vi "Harvest_Folder_Client.vi"(4 "Get all Server Files":bool, 5 "Check Updates on Server?":bool, 6 "Archive Files?":bool, 7 "Folder to Harvest":path=path "/Lacie_20/EnFlo_Data/Andrew_Burt/Results") -> (0 "error out":errorcluster, 1 "Folder contents changed?":bool, 2 "Files to Pull From Server":path[](array[path]), 3 "Files to Push to Server":path[](array[path]))   [LabVIEW 2013]
uses:
  Sub VIs/Harvest_Global.vi
  Anemometry/Anemometry Sub Vis/Globals/Preference_global.vi
  Anemometry/Anemometry Sub Vis/Globals/Constants_global.vi
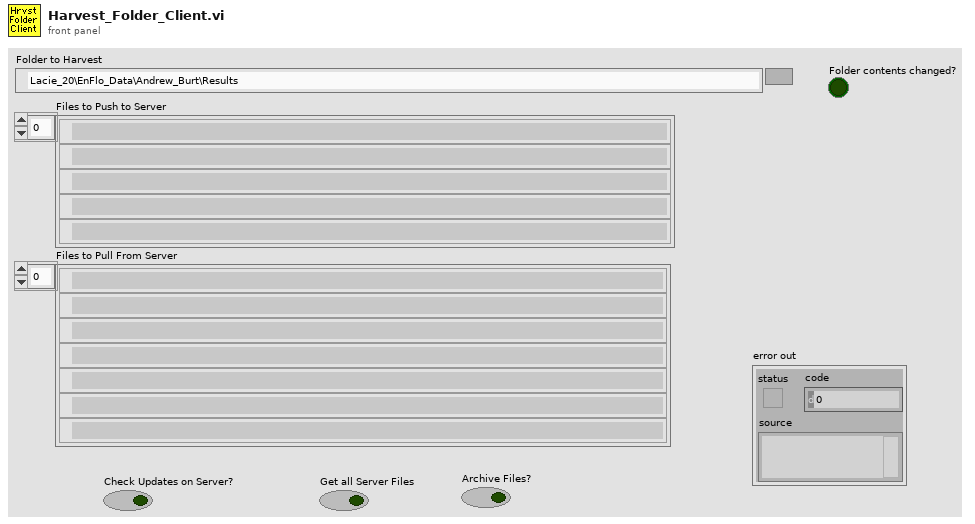
[diagram p1: front panel]
types:
  T1 = typedef "Server_Comms.ctl" = enum16{"Server Link Healthy", "Do Not Link To Server"}
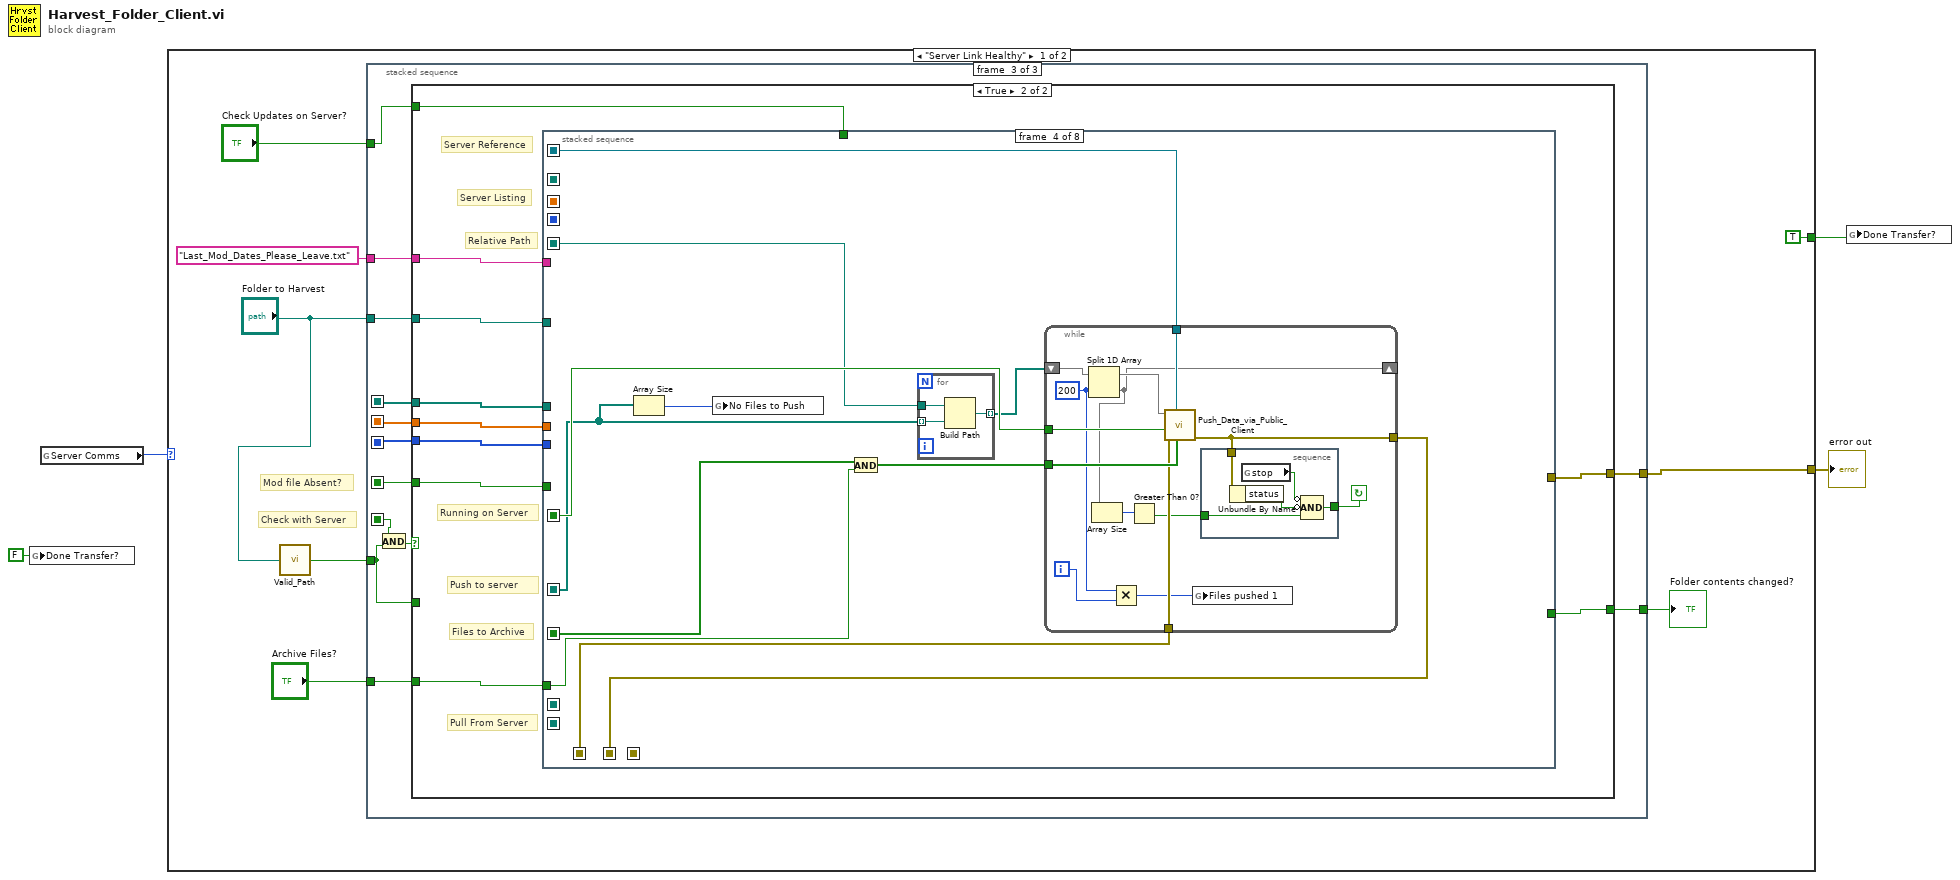
[diagram p0: block diagram]
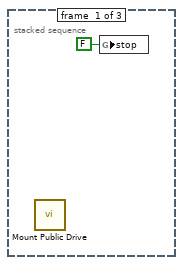
[diagram p2: hidden frame]
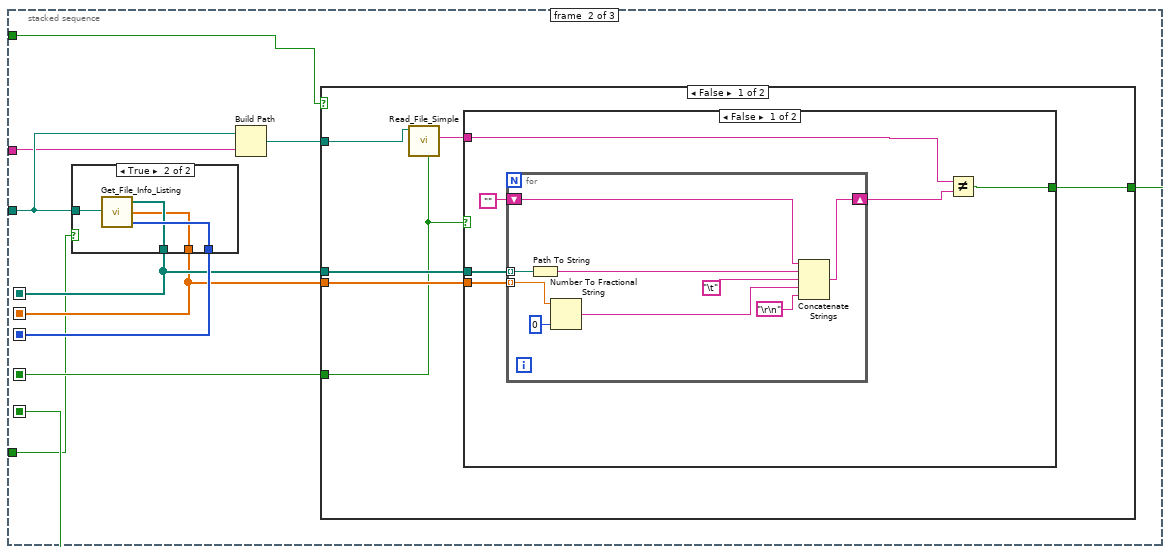
[diagram p3: hidden frame]
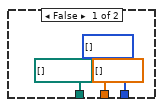
[diagram p4: hidden frame]
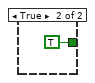
[diagram p5: hidden frame]
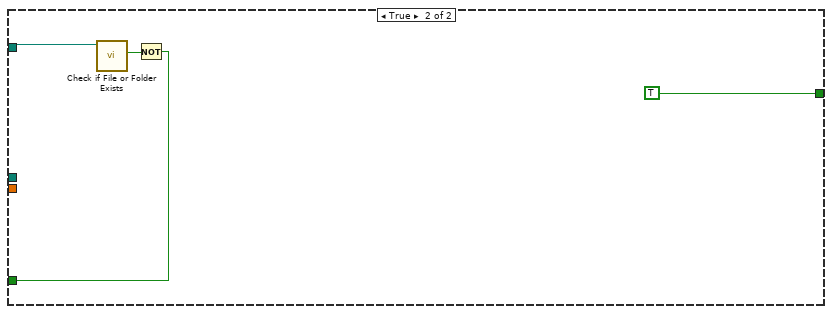
[diagram p6: hidden frame]
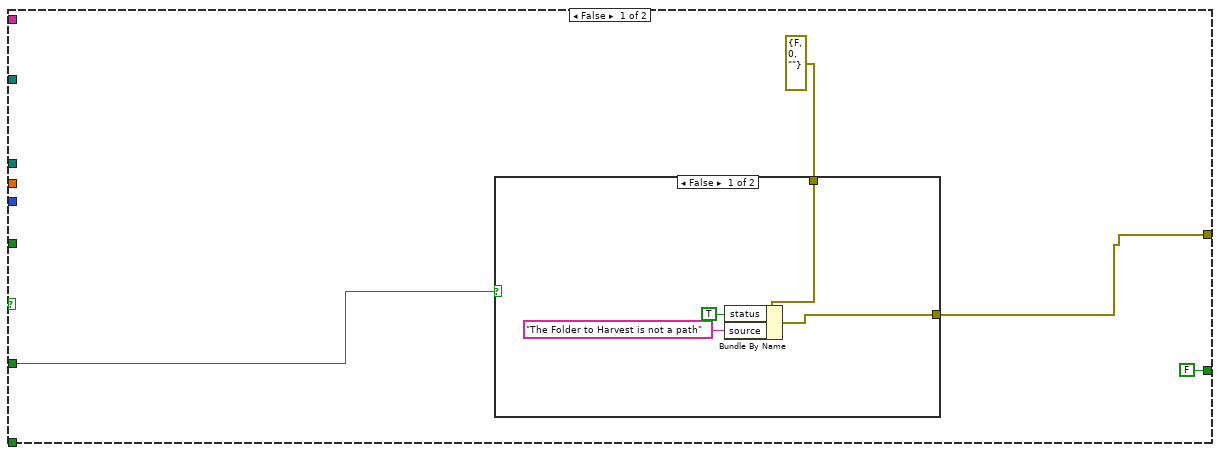
[diagram p7: hidden frame]
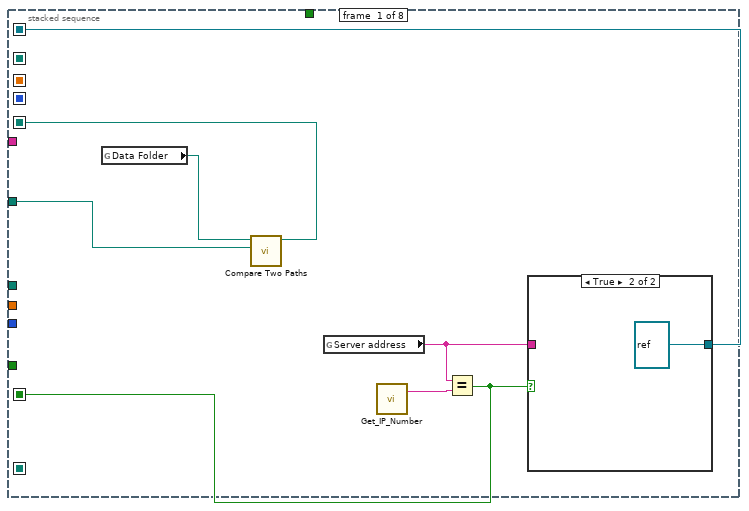
[diagram p9: hidden frame]
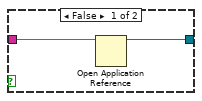
[diagram p10: hidden frame]
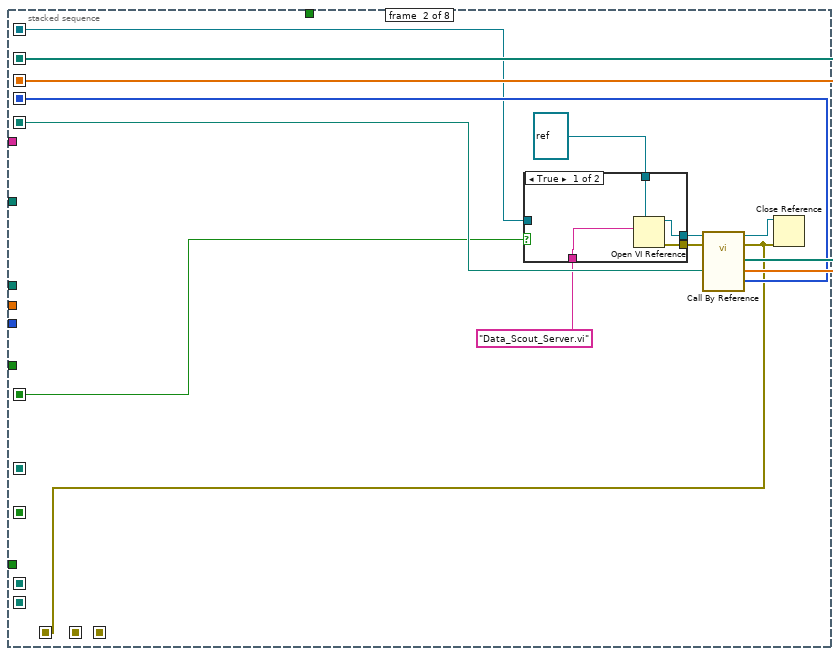
[diagram p11: hidden frame]
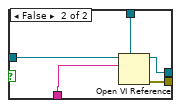
[diagram p12: hidden frame]
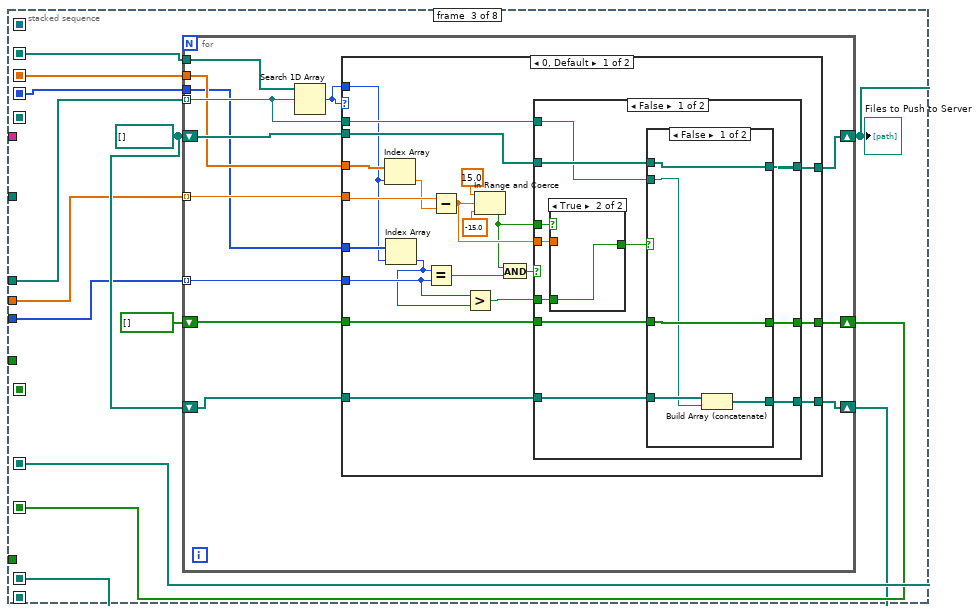
[diagram p13: hidden frame]
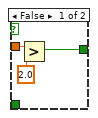
[diagram p14: hidden frame]
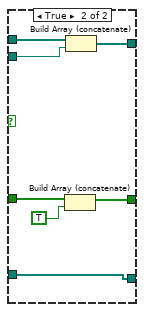
[diagram p15: hidden frame]
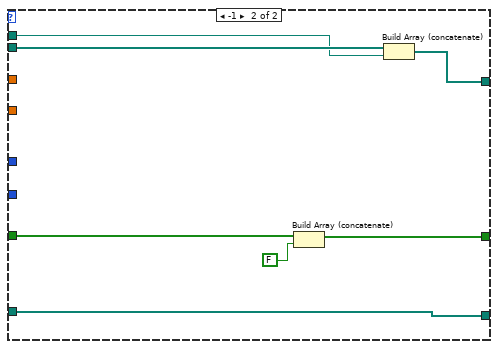
[diagram p17: hidden frame]
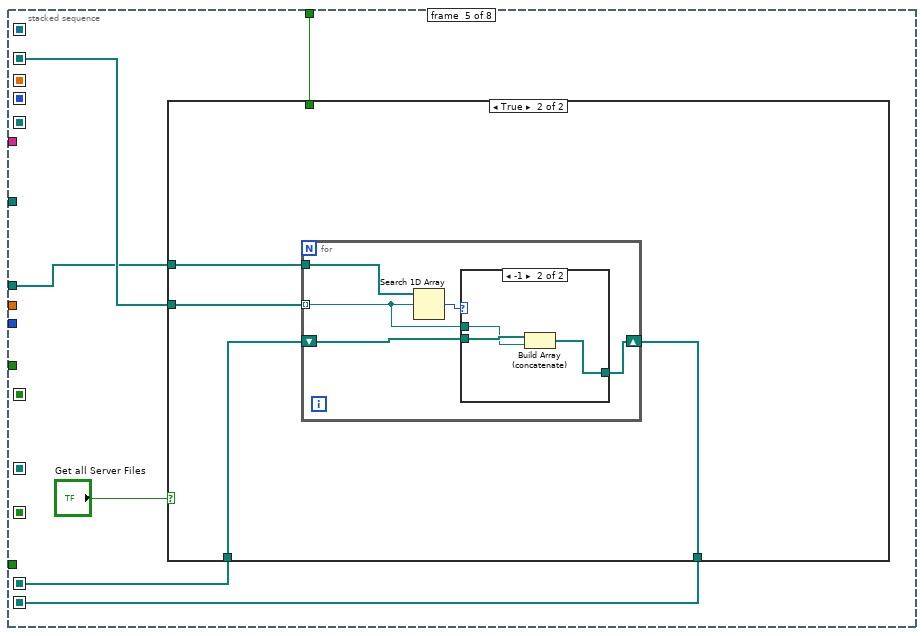
[diagram p18: hidden frame]
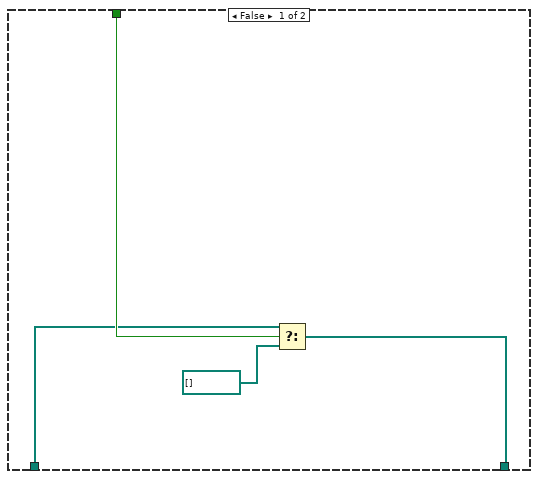
[diagram p19: hidden frame]
diagram:
  n1 = global write "Harvest_Global.vi" "Done Transfer?"(FALSE ("Done Transfer?")) -> ()
  n2 = global read "Preference_global.vi" "Server Comms"() -> (w4:T1)
  n3 = case shown="\"Server Link Healthy\"" w4 {
    tunnel: [w6 w324] -> w3
    tunnel: [TRUE ("Done Transfer?") TRUE ("Done Transfer?")] -> w1
    frame "Server Link Healthy" {
      # "Mod file Absent?"
      # "Check with Server"
      n4 = call "Valid_Path.vi"("Filename"="Folder to Harvest") -> ("Valid Path?"=w9:bool)
      n5 = stacked-sequence {
        seq-local: [_ w22 _] -> [_ _ w68]
        seq-local: [_ w21 _] -> [_ _ w67]
        seq-local: [_ w23 _] -> [_ _ w66]
        seq-local: [_ w20 _] -> [_ _ w61]
        seq-local: [_ w19 _] -> [_ _ w62]
        tunnel: "Folder to Harvest" -> [_ w18 w69]
        tunnel: "Last_Mod_Dates_Please_Leave.txt" ("name or relative path") -> [_ w17 w65]
        tunnel: [_ _ w64] -> w6
        tunnel: [_ _ w63] -> w11
        tunnel: w9 -> [_ w15 w59]
        tunnel: "Archive Files?" -> [_ _ w58]
        tunnel: "Check Updates on Server?" -> [_ w14 w57]
        frame #0 {
          n6 = call "Mount Public Drive.vi"() -> ()  [unwired: 12 in]
          n7 = global write "Harvest_Global.vi" "stop"(FALSE ("stop")) -> ()
        }
        frame #1 {
          n8 = case shown="True" w15 {
            tunnel: [i64[] [] ("Size") w30] -> w23
            tunnel: [path[] [] ("Path") w29] -> w22
            tunnel: [dbl[] [] ("Last Mod") w28] -> w21
            tunnel: w18 -> [_ w27]
            frame False {
            }
            frame True {
              n9 = call "Get_File_Info_Listing.vi"("path"=w27) -> ("Path"=w29:path[], "Last Mod"=w28:dbl[], "Size"=w30:i64[])
            }
          }
          n10 = Build Path(base path=w18, name or relative path=w17) -> (appended path=w16:path)
          n11 = case shown="False" w14 {
            tunnel: w22 -> [w36 _]
            tunnel: w21 -> [w35 _]
            tunnel: [w33 TRUE] -> w20
            tunnel: [w32 w53] -> w19
            tunnel: w16 -> [w31 w55]
            frame False {
              n12 = call "Read_File_Simple.vi"("Filename"=w31) -> ("Error?"=w32:bool, "string"=w34:string)  [unwired: 4 in, 4 out]
              n13 = case shown="False" w32 {
                tunnel: w36 -> [w41 _]
                tunnel: w35 -> [w40 _]
                tunnel: w34 -> [w39 _]
                tunnel: [w37 TRUE] -> w33
                frame False {
                  n14 = for {
                    tunnel: w41 -> [w51] mode=indexing
                    tunnel: w40 -> [w49] mode=indexing
                    shift-right: [w43] -> w38
                    shift-left: "" -> [w48]
                    n15 = Path To String(path=w51) -> (string=w47:string)
                    n16 = Number To Fractional String(number=w49, precision (6)=i16 0) -> (F-format string=w45:string)  [unwired: 2 in]
                    n17 = Concatenate Strings(w48, w47, "\t", w45, "\r\n") -> (w43:string)
                  }
                  n18 = Not Equal?(x=w39, y=w38) -> (x != y?=w37:bool)
                }
                frame True {
                }
              }
            }
            frame True {
              n19 = call <vilib>:"Check if File or Folder Exists.vi"("path"=w55) -> ("file or folder exists?"=w54:bool)  [unwired: 8 in, 2 out]
              n20 = Not(x=w54) -> (.not. x?=w53:bool)
            }
          }
        }
        frame #2 {
          n21 = And(x=w61, y=w59) -> (x .and. y?=w60:bool)
          n22 = case shown="True" w60 {
            tunnel: w69 -> [_ w88]
            tunnel: w68 -> [_ w87]
            tunnel: w67 -> [_ w86]
            tunnel: w66 -> [_ w85]
            tunnel: w65 -> [_ w84]
            tunnel: [w70 w83] -> w64
            tunnel: [FALSE w82] -> w63
            tunnel: w62 -> [_ w81]
            tunnel: w59 -> [w72 _]
            tunnel: w58 -> [_ w80]
            tunnel: w57 -> [_ w79]
            frame False {
              n23 = case shown="False" w72 {
                tunnel: errorcluster {"status"=FALSE, "code"=0, "source"=""} ("Error IO") -> [w77 w78]
                tunnel: [w74 w78] -> w70
                frame False {
                  n24 = Bundle By Name(cluster=w77, "status"=TRUE, "source"="The Folder to Harvest is not a path") -> (w74:errorcluster)
                }
                frame True {
                }
              }
            }
            frame True {
              # "Running on Server"
              # "Server Reference"
              # "Pull From Server"
              # "Server Listing"
              # "Relative Path"
              # "Files to Archive"
              # "Push to server"
              n25 = stacked-sequence {
                seq-local: [_ w107 _ _ _ _ _ _] -> [_ _ w130 _ w239 _ _ _]
                seq-local: [_ w106 _ _ _ _ _ _] -> [_ _ w129 _ _ _ _ _]
                seq-local: [_ _ w128 _ _ _ _ _] -> [_ _ _ w203 _ _ w299 _]
                seq-local: [_ _ w127 _ _ _ _ _] -> [_ _ _ w209 _ _ _ _]
                seq-local: [w93 _ _ _ _ _ _ _] -> [_ w108 _ w206 _ w266 _ _]
                seq-local: [_ w105 _ _ _ _ _ _] -> [_ _ w124 _ _ _ _ _]
                seq-local: [_ _ w123 _ _ _ _ _] -> [_ _ _ _ w238 _ _ _]
                seq-local: [w92 _ _ _ _ _ _ _] -> [_ w100 _ w211 _ w264 _ w319]
                seq-local: [_ w101 _ _ _ _ _ _] -> [_ _ _ w205 _ _ _ _]
                seq-local: [_ _ _ w210 _ _ _ _] -> [_ _ _ _ _ w261 _ _]
                seq-local: [_ _ _ _ w237 _ _ _] -> [_ _ _ _ _ w259 w298 _]
                seq-local: [_ _ _ _ _ w260 _ _] -> [_ _ _ _ _ _ w292 _]
                seq-local: [w89 _ _ _ _ _ _ _] -> [_ w99 _ w212 _ w263 _ w320]
                tunnel: w88 -> [w94 _ _ _ _ _ w294 _]
                tunnel: w87 -> [_ _ w122 _ w236 _ _ _]
                tunnel: w86 -> [_ _ w121 _ _ _ _ _]
                tunnel: w85 -> [_ _ w120 _ _ _ _ _]
                tunnel: w84 -> [_ _ _ _ _ _ w293 _]
                tunnel: [_ _ _ _ _ _ w292 _] -> w83
                tunnel: [_ _ _ _ _ _ w291 _] -> w82
                tunnel: w81 -> [_ _ _ _ _ _ w290 _]
                tunnel: w80 -> [_ _ _ w208 _ w262 _ _]
                tunnel: w79 -> [_ _ _ _ w235 _ _ _]
                frame #0 {
                  n26 = global read "Constants_global.vi" "Data Folder"() -> (w95:path)
                  n27 = call <vilib>:"Compare Two Paths.vi"("Path 2"=w94, "Path 1"=w95) -> ("Relative Path from 1 to 2"=w93:path)  [unwired: 6 in, 3 out]
                  n28 = global read "Preference_global.vi" "Server address"() -> (w91:string)
                  n29 = call "Get_IP_Number.vi"() -> ("IP Number"=w90:string)  [unwired: 1 out]
                  n30 = Equal?(x=w91, y=w90) -> (x = y?=w89:bool)
                  n31 = case shown="True" w89 {
                    tunnel: [w97 refnum<vi> refnum ("application reference (local)")] -> w92
                    tunnel: w91 -> [w96 _]
                    frame False {
                      n32 = Open Application Reference(11:w96) -> (3:w97:refnum<vi>)  [unwired: 2 in, 2 out]
                    }
                    frame True {
                    }
                  }
                }
                frame #1 {
                  n33 = case shown="True" w99 {
                    tunnel: [w114 w119] -> w110
                    tunnel: [w113 w118] -> w109
                    tunnel: "Data_Scout_Server.vi" -> [w112 w117]
                    tunnel: refnum<vi> refnum ("Scout Server") -> [w111 w116]
                    tunnel: w100 -> [_ w115]
                    frame True {
                      n34 = Open VI Reference(type specifier VI Refnum (for type only)=w111, vi path=w112) -> (vi reference=w114:refnum<vi>, error out=w113:errorcluster)  [unwired: 2 in, 2 out]
                    }
                    frame False {
                      n35 = Open VI Reference(type specifier VI Refnum (for type only)=w116, application reference (local)=w115, vi path=w117) -> (vi reference=w119:refnum<vi>, error out=w118:errorcluster)  [unwired: 1 in, 2 out]
                    }
                  }
                  n36 = call-by-ref "?"(reference=w110, error in=w109, "Relative Path"=w108) -> (reference out=w104:refnum<vi>, error out=w101:errorcluster, "Path"=w107:path[], "Last Mod"=w106:dbl[], "Size"=w105:i64[])
                  n37 = Close Reference(reference=w104, error in (no error)=w101) -> ()  [unwired: 1 out]
                }
                frame #2 {
                  w125 = path[] []
                  n38 = for {
                    tunnel: w122 -> [w142] mode=indexing
                    shift-right: [w131] -> w128
                    shift-left: w125 -> [w143]
                    tunnel: w130 -> [w141]
                    tunnel: w129 -> [w139]
                    tunnel: w121 -> [w138] mode=indexing
                    shift-right: [w136] -> w127
                    shift-left: bool[] [] -> [w137]
                    shift-right: [w134] -> w123
                    shift-left: w125 -> [w135]
                    tunnel: w124 -> [w133]
                    tunnel: w120 -> [w132] mode=indexing
                    n39 = Search 1D Array(1D array=w141, element=w142) -> (index of element=w140:i32)  [unwired: 1 in]
                    n40 = case shown="0, Default" w140 {
                      tunnel: w143 -> [w162 w201]
                      tunnel: [w163 w200] -> w131
                      tunnel: w142 -> [w161 w199]
                      tunnel: w140 -> [w150 _]
                      tunnel: w139 -> [w164 _]
                      tunnel: w138 -> [w160 _]
                      tunnel: w137 -> [w155 w198]
                      tunnel: [w154 w197] -> w136
                      tunnel: w135 -> [w153 w195]
                      tunnel: [w152 w195] -> w134
                      tunnel: w133 -> [w151 _]
                      tunnel: w132 -> [w148 _]
                      frame 0, Default {
                        n41 = Index Array(array=w164, index=w150) -> (element=w159:dbl)
                        n42 = Index Array(array=w151, index=w150) -> (element=w147:i64)
                        n43 = Equal?(x=w147, y=w148) -> (x = y?=w146:bool)
                        n44 = Subtract(x=w160, y=w159) -> (x-y=w156:dbl)
                        n45 = Greater?(x=w148, y=w147) -> (0:w145:bool)
                        n46 = In Range and Coerce(upper limit=15.0, x=w156, lower limit=-15.0) -> (In Range?=w144:bool)  [unwired: 1 out]
                        n47 = And(x=w144, y=w146) -> (x .and. y?=w149:bool)
                        n48 = case shown="False" w149 {
                          tunnel: [w174 w194] -> w163
                          tunnel: w162 -> [w173 w194]
                          tunnel: w161 -> [w172 _]
                          tunnel: w156 -> [w171 _]
                          tunnel: w155 -> [w170 w193]
                          tunnel: [w169 w193] -> w154
                          tunnel: w153 -> [w168 w192]
                          tunnel: [w167 w192] -> w152
                          tunnel: w145 -> [w166 _]
                          tunnel: w144 -> [w165 _]
                          frame False {
                            n49 = case shown="True" w165 {
                              tunnel: [w178 w179] -> w175
                              tunnel: w171 -> [w177 _]
                              tunnel: w166 -> [_ w179]
                              frame False {
                                n50 = Greater?(x=w177, y=2.0) -> (0:w178:bool)
                              }
                              frame True {
                              }
                            }
                            n51 = case shown="False" w175 {
                              tunnel: [w184 w191] -> w174
                              tunnel: w173 -> [w184 w190]
                              tunnel: w172 -> [w180 w187]
                              tunnel: w170 -> [w183 w189]
                              tunnel: [w183 w188] -> w169
                              tunnel: w168 -> [w182 w185]
                              tunnel: [w181 w185] -> w167
                              frame False {
                                n52 = Build Array (concatenate)(w182, w180) -> (w181:path[])
                              }
                              frame True {
                                n53 = Build Array (concatenate)(w189, TRUE) -> (w188:bool[])
                                n54 = Build Array (concatenate)(w190, w187) -> (w191:path[])
                              }
                            }
                          }
                          frame True {
                          }
                        }
                      }
                      frame -1 {
                        n55 = Build Array (concatenate)(w198, FALSE) -> (w197:bool[])
                        n56 = Build Array (concatenate)(w201, w199) -> (w200:path[])
                      }
                    }
                  }
                  "Files to Push to Server" <- w128
                }
                frame #3 {
                  n57 = Array Size(array=w203) -> (size(s)=w202:i32)
                  n58 = global write "Harvest_Global.vi" "No Files to Push"(w202) -> ()
                  n59 = And(x=w209, y=w208) -> (x .and. y?=w207:bool[])
                  n60 = for {
                    tunnel: w206 -> [w234]
                    tunnel: w203 -> [w233] mode=indexing
                    tunnel: [w232] -> w204 mode=indexing
                    n61 = Build Path(base path=w234, name or relative path=w233) -> (appended path=w232:path)
                  }
                  n62 = while {
                    tunnel: w212 -> [w226]
                    tunnel: w211 -> [w225]
                    tunnel: [w218] -> w210
                    tunnel: w207 -> [w224]
                    tunnel: w205 -> [w223]
                    shift-right: [w220] -> _
                    shift-left: w204 -> [w222]
                    i -> [w214]
                    stop <- w216 continue-if-true
                    w213 = 200 ("index")
                    n63 = Split 1D Array(array=w222, index=w213) -> (first subarray=w221:path[], second subarray=w220:path[])
                    n64 = Array Size(array=w220) -> (size(s)=w219:i32)
                    n65 = Multiply(x=w213, y=w214) -> (x*y=w215:i32)
                    n66 = Greater Than 0?(x=w219) -> (x > 0?=w217:bool)
                    n67 = call "Push_Data_via_Public_Client.vi"("Archive File?"=w224, "application reference"=w225, "error in (no error)"=w223, "Running on Server?"=w226, "Path of Files relative to EnFlo Data Root"=w221) -> ("error out"=w218:errorcluster)  [unwired: 5 in]
                    n68 = global write "Harvest_Global.vi" "Files pushed 1"(w215) -> ()
                    n69 = stacked-sequence {
                      tunnel: w218 -> [w231]
                      tunnel: w217 -> [w229]
                      tunnel: [w228] -> w216
                      frame #0 {
                        n70 = Unbundle By Name(w231) -> ("status"=w230:bool)
                        n71 = global read "Harvest_Global.vi" "stop"() -> (w227:bool)
                        n72 = Compound Arithmetic op=AND(invert w227, invert w230, w229) -> (w228:bool)
                      }
                    }
                  }
                }
                frame #4 {
                  n73 = case shown="True" "Get all Server Files" {
                    tunnel: w236 -> [_ w248]
                    tunnel: w239 -> [_ w247]
                    tunnel: w238 -> [w243 w246]
                    tunnel: [w242 w245] -> w237
                    tunnel: w235 -> [w244 _]
                    frame False {
                      n74 = Select(t=w243, s=w244, f=path[] []) -> (s? t:f=w242:path[])
                    }
                    frame True {
                      n75 = for {
                        tunnel: w247 -> [w252] mode=indexing
                        shift-right: [w249] -> w245
                        shift-left: w246 -> [w253]
                        tunnel: w248 -> [w251]
                        n76 = Search 1D Array(1D array=w251, element=w252) -> (index of element=w250:i32)  [unwired: 1 in]
                        n77 = case shown="-1" w250 {
                          tunnel: w253 -> [w254 w257]
                          tunnel: [w254 w256] -> w249
                          tunnel: w252 -> [_ w255]
                          frame 0, Default {
                          }
                          frame -1 {
                            n78 = Build Array (concatenate)(w257, w255) -> (w256:path[])
                          }
                        }
                      }
                    }
                  }
                }
                frame #5 {
                  n79 = Array Size(array=w259) -> (size(s)=w258:i32)
                  n80 = for {
                    tunnel: w266 -> [w288]
                    tunnel: w259 -> [w287] mode=indexing
                    tunnel: [w286] -> w265 mode=indexing
                    n81 = Build Path(base path=w288, name or relative path=w287) -> (appended path=w286:path)
                  }
                  n82 = global write "Harvest_Global.vi" "No Files to Pull"(w258) -> ()
                  n83 = while {
                    tunnel: [w275] -> w260
                    shift-right: [w279] -> _
                    shift-left: w265 -> [w280]
                    tunnel: w264 -> [w273]
                    tunnel: w263 -> [w272]
                    tunnel: w262 -> [w271]
                    tunnel: w261 -> [w270]
                    i -> [w269]
                    stop <- w276 continue-if-true
                    w268 = 200 ("index")
                    n84 = Multiply(x=w268, y=w269) -> (x*y=w267:i32)
                    n85 = Split 1D Array(array=w280, index=w268) -> (first subarray=w274:path[], second subarray=w279:path[])
                    n86 = global write "Harvest_Global.vi" "Files Pulled 1"(w267) -> ()
                    n87 = Array Size(array=w279) -> (size(s)=w278:i32)
                    n88 = call "Pull_Data_via_Public_Client.vi"("application reference"=w273, "error in (no error)"=w270, "Archive Files?"=w271, "Running on Server?"=w272, "Path of File relative to EnFlo Data Root"=w274) -> ("error out"=w275:errorcluster)  [unwired: 1 in]
                    n89 = Greater Than 0?(x=w278) -> (x > 0?=w277:bool)
                    n90 = stacked-sequence {
                      tunnel: w277 -> [w284]
                      tunnel: [w283] -> w276
                      tunnel: w275 -> [w282]
                      frame #0 {
                        n91 = Unbundle By Name(w282) -> ("status"=w285:bool)
                        n92 = global read "Harvest_Global.vi" "stop"() -> (w281:bool)
                        n93 = Compound Arithmetic op=AND(invert w281, invert w285, w284) -> (w283:bool)
                      }
                    }
                  }
                  "Files to Pull From Server" <- w259
                }
                frame #6 {
                  n94 = Array Size(array=w298) -> (size(s)=w296:i32)
                  n95 = Array Size(array=w299) -> (size(s)=w297:i32)
                  n96 = Add(x=w297, y=w296) -> (x+y=w295:i32)
                  n97 = Greater Than 0?(x=w295) -> (x > 0?=w291:bool)
                  n98 = Or(x=w290, y=w291) -> (x .or. y?=w289:bool)
                  n99 = case shown="No Error" w292 {
                    tunnel: w294 -> [w302 _]
                    tunnel: w293 -> [w301 _]
                    tunnel: w289 -> [w300 _]
                    frame No Error {
                      n100 = case shown="True" w300 {
                        tunnel: w302 -> [_ w305]
                        tunnel: w301 -> [_ w303]
                        frame False {
                        }
                        frame True {
                          n101 = call "Get_File_Info_Listing.vi"("path"=w305) -> ("Path"=w309:path[], "Last Mod"=w308:dbl[])  [unwired: 1 out]
                          n102 = for {
                            tunnel: w309 -> [w318] mode=indexing
                            tunnel: w308 -> [w316] mode=indexing
                            shift-right: [w310] -> w306
                            shift-left: "" -> [w315]
                            n103 = Path To String(path=w318) -> (string=w314:string)
                            n104 = Number To Fractional String(number=w316, precision (6)=i16 0) -> (F-format string=w312:string)  [unwired: 2 in]
                            n105 = Concatenate Strings(w315, w314, "\t", w312, "\r\n") -> (w310:string)
                          }
                          n106 = Build Path(base path=w305, name or relative path=w303) -> (appended path=w304:path)
                          n107 = call "Write_File_Simple.vi"("character string"=w306, "file path"=w304) -> ()  [unwired: 1 in, 2 out]
                        }
                      }
                    }
                    frame Error {
                    }
                  }
                }
                frame #7 {
                  n108 = case shown="False" w320 {
                    tunnel: w319 -> [w321 _]
                    frame False {
                      n109 = Close Reference(reference=w321) -> ()  [unwired: 1 in, 1 out]
                    }
                    frame True {
                    }
                  }
                }
              }
            }
          }
        }
      }
      "Folder contents changed?" <- w11
    }
    frame "Do Not Link To Server" {
      n110 = Bundle By Name(cluster=errorcluster {"status"=FALSE, "code"=0, "source"=""} ("Error IO"), "status"=TRUE, "source"="Preference Panel set to \"Do Not Link To Server\"") -> (w324:errorcluster)
    }
  }
  "error out" <- w3
  n111 = global write "Harvest_Global.vi" "Done Transfer?"(w1) -> ()
